vi "m1m3_putSample_IMSData.vi"(8 "error in (no error)":errorcluster, 11 "IMSData_Ctl":T1={"Timestamp"=0.0, "RawSensorData[8]"=[0.0, 0.0, 0.0, 0.0, 0.0, 0.0, 0.0, 0.0], "XPosition"=0.0, "YPosition"=0.0, "ZPosition"=0.0, "XRotation"=0.0, "YRotation"=0.0, "ZRotation"=0.0}) -> (0 "error out":errorcluster, 2 "function return":i32, 3 "IMSData_Ctl out":T1)   [LabVIEW 2016, in "SALLV_m1m3.lvlib"]
doc: "int m1m3_shm_putSample_IMSDataLV(m1m3_IMSDataLV *IMSData_Ctl );"
uses:
  SALLV_m1m3.lvlib
  DataTypes/IMSData.ctl
  SALLV_m1m3.so
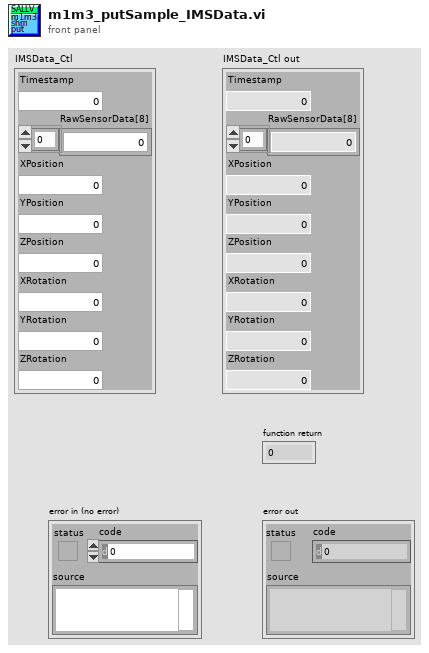
[diagram p1: front panel]
types:
  T1 = typedef "SALLV_m1m3.lvlib/IMSData.ctl" = cluster{"Timestamp":dbl, "RawSensorData[8]":sgl[], "XPosition":sgl, "YPosition":sgl, "ZPosition":sgl, "XRotation":sgl, "YRotation":sgl, "ZRotation":sgl}
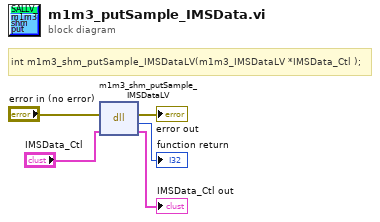
[diagram p0: block diagram]
diagram:
  # "int m1m3_shm_putSample_IMSDataLV(m1m3_IMSDataLV *IMSData_Ctl );"
  n1 = dll-call lib="opt/CODE/SALLV_m1m3/SALLV_m1m3.*" fn="m1m3_shm_putSample_IMSDataLV"(error in="error in (no error)", "IMSData_Ctl"="IMSData_Ctl") -> (error out=→"error out":errorcluster, →"function return":i32, "IMSData_Ctl"=→"IMSData_Ctl out":T1)  [unwired: 2 in, 1 out]
